vi "FTT Display.vi"(8 "error in (no error)":errorcluster, 10 "Mode":enum16{"Read", "Write"}(ring), 11 "Display":T1) -> (0 "error out":errorcluster, 3 "Display out":T1)   [LabVIEW 2014]
uses:
  Type'def/FTT Display Type.ctl
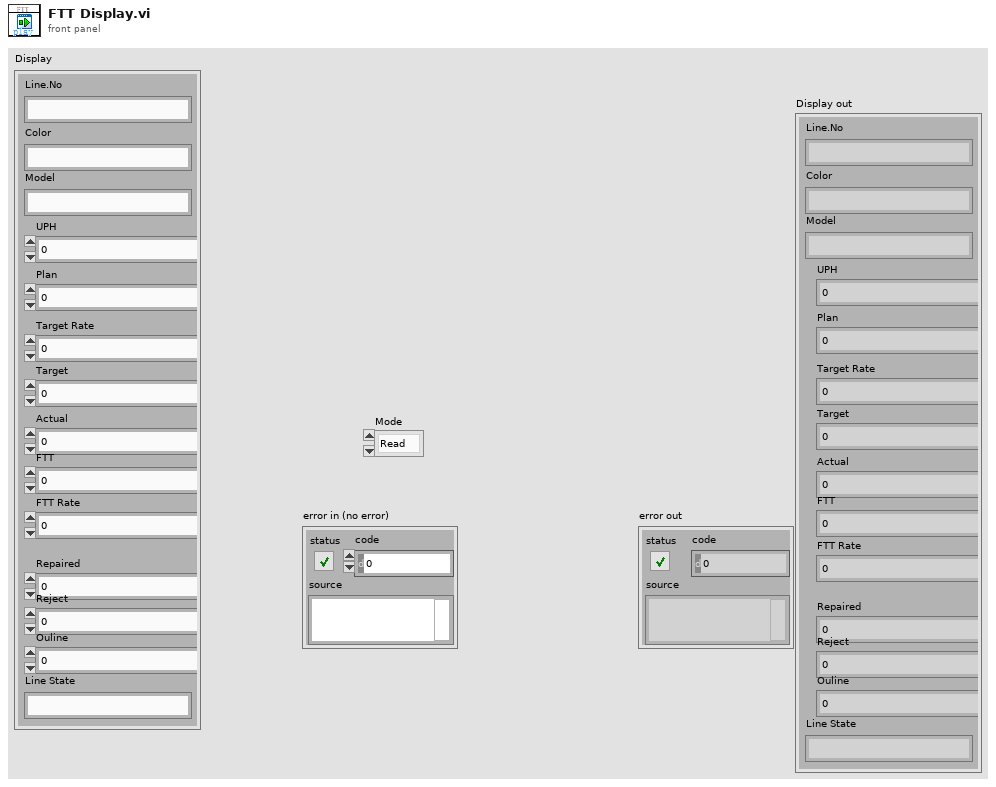
[diagram p1: front panel]
types:
  T1 = typedef "FTT Display Type.ctl" = cluster{"Line.No":string, "Model":string, "Color":string, "UPH":dbl, "Plan":dbl, "Target Rate":dbl, "Target ":dbl, "Actual":dbl, "FTT":dbl, "FTT Rate":dbl, "Repaired":dbl, "Reject":dbl, "Ouline":dbl, "Line State":string}
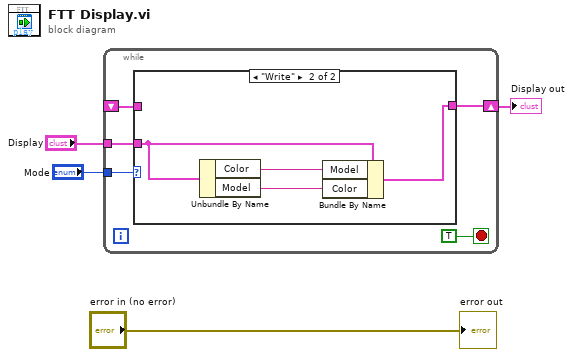
[diagram p0: block diagram]
diagram:
  n1 = while {
    tunnel: "Mode" -> [w8]
    tunnel: "Display" -> [w7]
    shift-right: [w6] -> w1
    shift-left: _ -> [w5]
    stop <- TRUE stop-if-true
    n2 = case shown="\"Write\"" w8 {
      tunnel: w7 -> [_ w14]
      tunnel: [w10 w11] -> w6
      tunnel: w5 -> [w10 _]
      frame "Read", Default {
      }
      frame "Write" {
        n3 = Unbundle By Name(w14) -> ("Color"=w13:string, "Model"=w12:string)
        n4 = Bundle By Name(cluster=w14, "Model"=w13, "Color"=w12) -> (w11:T1)
      }
    }
  }
  "Display out" <- w1
  "error out" <- "error in (no error)"
